vi "Run_Core.vi"(0 "Message Popup in":refnum<class "Numeric Functions.lvclass">, 11 "error in (no error)":errorcluster) -> (4 "Message Popup out":refnum<class "Numeric Functions.lvclass">, 6 "Return":variant, 15 "error out":errorcluster)   [LabVIEW 2019, in "Numeric Functions.lvclass"]
uses:
  Numeric Functions.lvclass
  Numeric Functions.lvclass/Numeric Functions.ctl
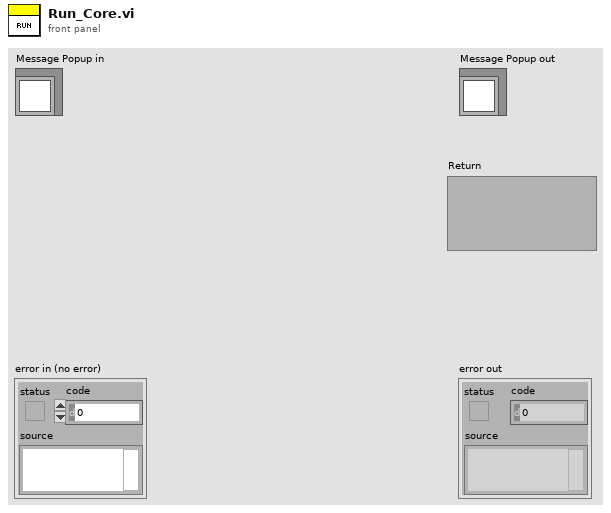
[diagram p1: front panel]
types:
  T1 = typedef "Numeric Functions.lvclass/Function List.ctl" = enum16{"Add", "Sub", "Multiply", "Divide", "Modulus", "Increament", "Decrement", "Square Root", "Square", "Negate", "Reciprocal", "Random Number", "Exponent", "Floor Division"}
  T2 = typedef "Datatype.ctl" = enum16{"Null", "Numeric", "String", "Bool", "Numeric 1D", "String 1D", "Bool 1D", "Numeric 2D", "String 2D", "Bool 2D", "Variant"}
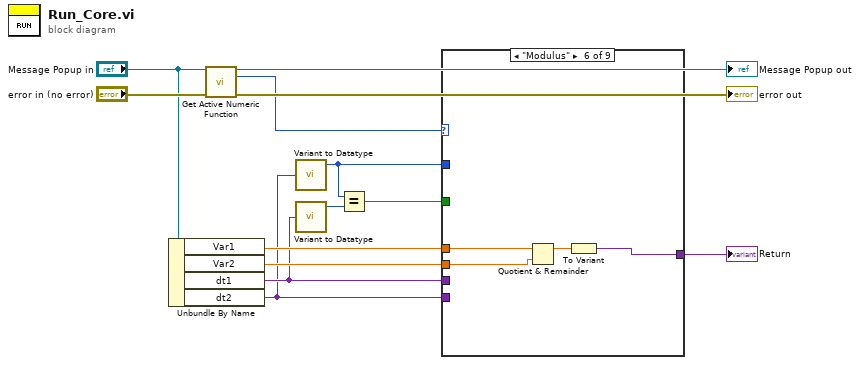
[diagram p0: block diagram]
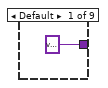
[diagram p2: hidden frame]
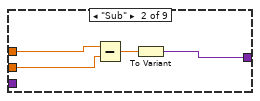
[diagram p3: hidden frame]
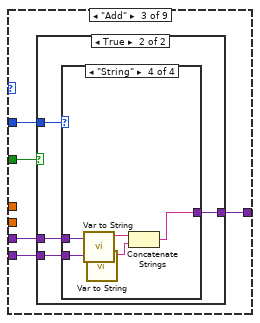
[diagram p4: hidden frame]
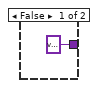
[diagram p5: hidden frame]
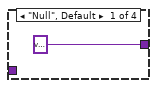
[diagram p6: hidden frame]
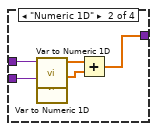
[diagram p7: hidden frame]
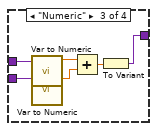
[diagram p8: hidden frame]
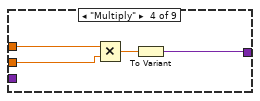
[diagram p9: hidden frame]
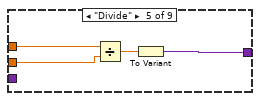
[diagram p10: hidden frame]
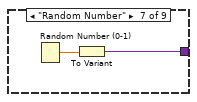
[diagram p11: hidden frame]
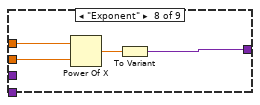
[diagram p12: hidden frame]
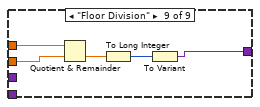
[diagram p13: hidden frame]
diagram:
  n1 = Unbundle By Name("Message Popup in") -> ("Var1"=w13:dbl, "Var2"=w12:dbl, "dt1"=w5:variant, "dt2"=w4:variant)
  n2 = call "Get Active Numeric Function.vi"("Numeric Functions in"="Message Popup in", "error in (no error)"="error in (no error)") -> ("Numeric Functions out"=→"Message Popup out":refnum<class "Numeric Functions.lvclass">, "Function"=w6:T1, "error out"=→"error out":errorcluster)  [unwired: 11 in]
  n3 = call "Variant to Datatype.vi"("Variant"=w4) -> ("Datatype"=w2:T2)  [unwired: 2 in, 2 out]
  n4 = call "Variant to Datatype.vi"("Variant"=w5) -> ("Datatype"=w3:T2)  [unwired: 2 in, 2 out]
  n5 = Equal?(x=w2, y=w3) -> (x = y?=w1:bool)
  n6 = case shown="\"Modulus\"" w6 {
    tunnel: w13 -> [_ w18 _ w49 w53 w57 _ w63 w68]
    tunnel: w12 -> [_ w17 _ w48 w52 w56 _ w62 w67]
    tunnel: [variant ("Variant") w15 w20 w46 w50 w55 w58 w60 w64] -> w11
    tunnel: w5 -> [_ _ w23 _ _ _ _ _ _]
    tunnel: w4 -> [_ _ w22 _ _ _ _ _ _]
    tunnel: w2 -> [_ _ w21 _ _ _ _ _ _]
    tunnel: w1 -> [_ _ w19 _ _ _ _ _ _]
    frame Default {
    }
    frame "Sub" {
      n7 = Subtract(x=w18, y=w17) -> (x-y=w16:dbl)
      n8 = To Variant(anything=w16) -> (Variant=w15:variant)
    }
    frame "Add" {
      n9 = case shown="True" w19 {
        tunnel: w23 -> [_ w28]
        tunnel: w22 -> [_ w27]
        tunnel: w21 -> [_ w26]
        tunnel: [variant ("Variant") w25] -> w20
        frame False {
        }
        frame True {
          n10 = case shown="\"String\"" w26 {
            tunnel: w28 -> [_ w34 w38 w45]
            tunnel: w27 -> [_ w33 w37 w44]
            tunnel: [variant ("Variant") w30 w35 w41] -> w25
            frame "Null", Default {
            }
            frame "Numeric 1D" {
              n11 = call "Var to Numeric 1D.vi"("Variant"=w34) -> ("Numeric Array"=w32:dbl[])  [unwired: 10 in]
              n12 = call "Var to Numeric 1D.vi"("Variant"=w33) -> ("Numeric Array"=w31:dbl[])  [unwired: 10 in]
              n13 = Add(x=w32, y=w31) -> (x+y=w30:dbl[])
            }
            frame "Numeric" {
              n14 = call "Var to Numeric.vi"("Variant"=w38) -> ("Numeric"=w40:dbl)  [unwired: 10 in]
              n15 = call "Var to Numeric.vi"("Variant"=w37) -> ("Numeric"=w39:dbl)  [unwired: 10 in]
              n16 = Add(x=w40, y=w39) -> (x+y=w36:dbl)
              n17 = To Variant(anything=w36) -> (Variant=w35:variant)
            }
            frame "String" {
              n18 = call "Var to String.vi"("Variant"=w45) -> ("String"=w43:string)  [unwired: 10 in]
              n19 = call "Var to String.vi"("Variant"=w44) -> ("String"=w42:string)  [unwired: 10 in]
              n20 = Concatenate Strings(w43, w42) -> (w41:string)
            }
          }
        }
      }
    }
    frame "Multiply" {
      n21 = Multiply(x=w49, y=w48) -> (x*y=w47:dbl)
      n22 = To Variant(anything=w47) -> (Variant=w46:variant)
    }
    frame "Divide" {
      n23 = Divide(x=w53, y=w52) -> (x/y=w51:dbl)
      n24 = To Variant(anything=w51) -> (Variant=w50:variant)
    }
    frame "Modulus" {
      n25 = Quotient & Remainder(x=w57, y=w56) -> (x-y*floor(x/y)=w54:dbl)  [unwired: 1 out]
      n26 = To Variant(anything=w54) -> (Variant=w55:variant)
    }
    frame "Random Number" {
      n27 = Random Number (0-1)() -> (number: 0 to 1=w59:dbl)
      n28 = To Variant(anything=w59) -> (Variant=w58:variant)
    }
    frame "Exponent" {
      n29 = Power Of X(1:w62, 2:w63) -> (0:w61:dbl)
      n30 = To Variant(anything=w61) -> (Variant=w60:variant)
    }
    frame "Floor Division" {
      n31 = Quotient & Remainder(x=w68, y=w67) -> (floor(x/y)=w66:dbl)  [unwired: 1 out]
      n32 = To Long Integer(number=w66) -> (32bit integer=w65:i32)
      n33 = To Variant(anything=w65) -> (Variant=w64:variant)
    }
  }
  "Return" <- w11
